vi "FiberSpectrograph_salCommander_enterControl.vi"(8 "error in (no error)":errorcluster) -> (0 "error out":errorcluster, 3 "function return":i32)   [LabVIEW 2016, in "SALLV_FiberSpectrograph.lvlib"]
doc: "int FiberSpectrograph_shm_salCommander_enterControlLV();"
uses:
  SALLV_FiberSpectrograph.lvlib
  SALLV_FiberSpectrograph.so
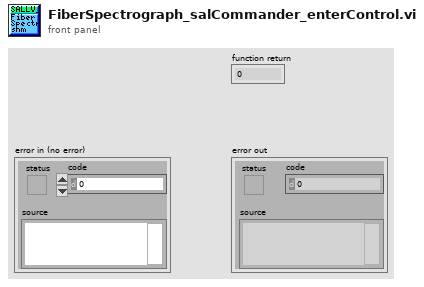
[diagram p1: front panel]
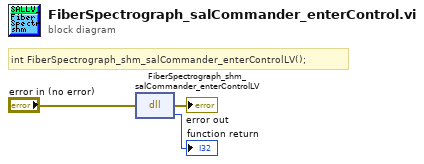
[diagram p0: block diagram]
diagram:
  # "int FiberSpectrograph_shm_salCommander_enterControlLV();"
  n1 = dll-call lib="home/harini/tcs/SALLV_FiberSpectrometer/SALLV_FiberSpectrograph.*" fn="FiberSpectrograph_shm_salCommander_enterControlLV"(error in="error in (no error)") -> (error out=→"error out":errorcluster, →"function return":i32)  [unwired: 2 in, 1 out]
